vi "Init.vi"(8 "error in (no error)":errorcluster, 11 "Icon Decorator In":refnum<class "Icon Decorator.lvclass">) -> (0 "error out":errorcluster, 3 "Icon Decorator Out":refnum<class "Icon Decorator.lvclass">)   [LabVIEW 2020, in "Icon Decorator.lvclass"]
uses:
  Icon Decorator.lvclass
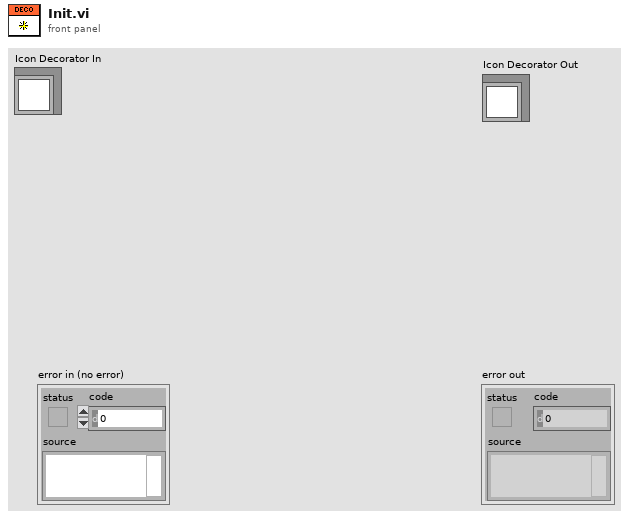
[diagram p1: front panel]
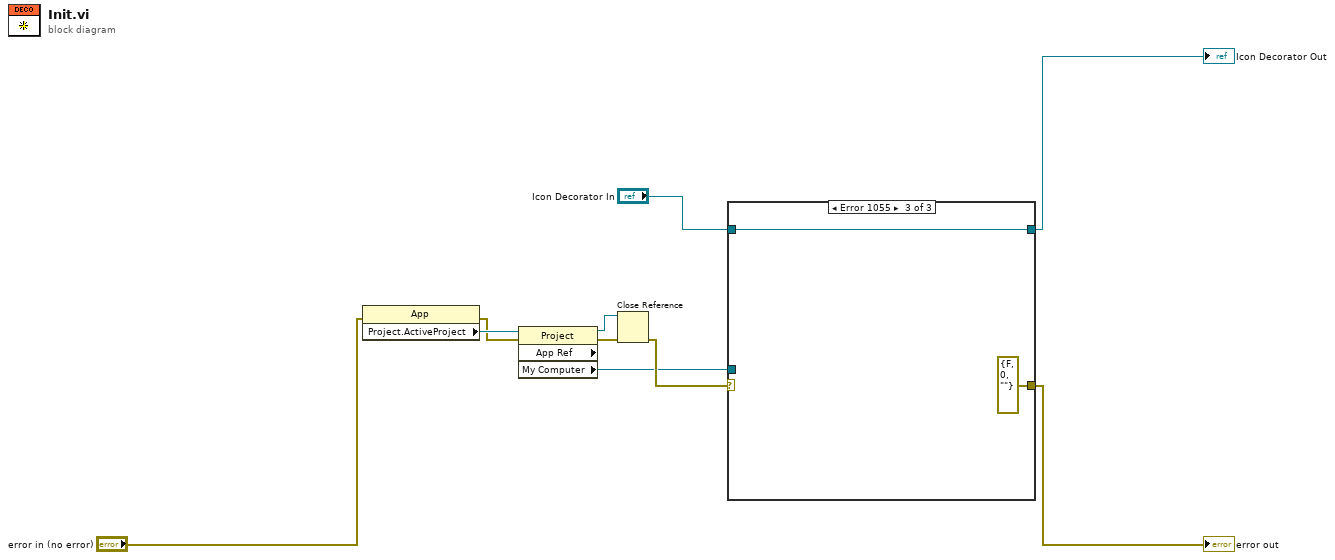
[diagram p0: block diagram]
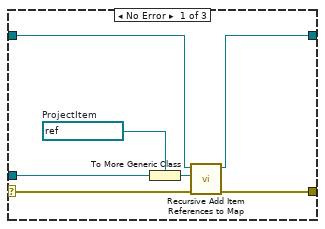
[diagram p2: hidden frame]
diagram:
  n1 = property class="App"(error in="error in (no error)") -> (error out=w5:errorcluster, "Project.ActiveProject"=w8:refnum<vi>)  [unwired: 1 in, 1 out]
  n2 = property class="Project" props=["App Ref", "My Computer"](reference=w8, error in=w5) -> (reference out=w6:refnum<vi>, error out=w7:errorcluster, "My Computer"=w9:refnum<vi>)  [unwired: 1 out]
  n3 = Close Reference(reference=w6, error in (no error)=w7) -> (error out=w10:errorcluster)
  n4 = case shown="Error 1055" w10 {
    selector: w10 -> [w13 w19 _]
    tunnel: "Icon Decorator In" -> [w17 w18 w21]
    tunnel: [w14 w18 w21] -> w3
    tunnel: w9 -> [w12 _ _]
    tunnel: [w11 w19 errorcluster {"status"=FALSE, "code"=0, "source"=""} ("error out")] -> w2
    frame No Error {
      w15 = refnum<vi> refnum  # ProjectItem
      n5 = To More Generic Class(target class=w15, reference=w12) -> (generic class reference=w16:refnum<vi>)
      n6 = call "Recursive Add Item References to Map.vi"("error in (no error)"=w13, "ProjectItem Refnum"=w16, "Icon Decorator In"=w17) -> ("error out"=w11:errorcluster, "Icon Decorator Out"=w14:refnum<class "Icon Decorator.lvclass">)  [unwired: 7 in]
    }
    frame Default {
    }
    frame Error {
    }
  }
  "error out" <- w2
  "Icon Decorator Out" <- w3
